vi "DRV_SDSU_reset_ctrler.vi"(0 "fd":i32, 11 "error in (no error)":errorcluster) -> (4 "fd out":i32, 8 "return value":i32, 15 "error out":errorcluster)   [LabVIEW 2016]
doc: "This VI resets the SDSU-II controller."
uses:
  c/lib/libarcDHE.so
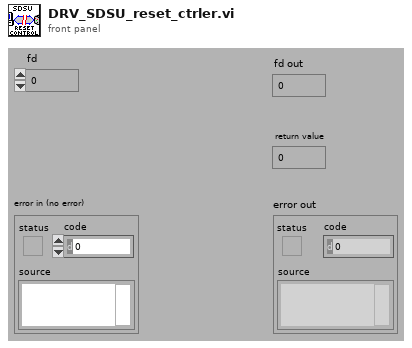
[diagram p1: front panel]
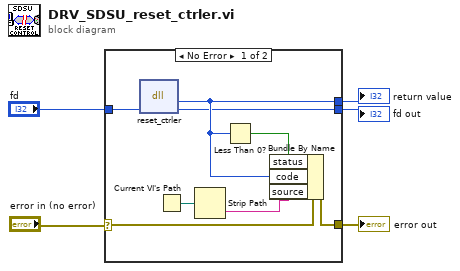
[diagram p0: block diagram]
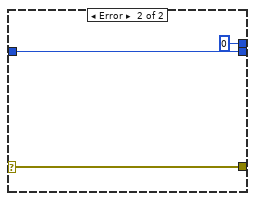
[diagram p2: hidden frame]
diagram:
  n1 = case shown="No Error" "error in (no error)" {
    selector: "error in (no error)" -> [w6 w14]
    tunnel: "fd" -> [w13 w16]
    tunnel: [w11 0] -> w4
    tunnel: [w8 w14] -> w3
    tunnel: [w7 w16] -> w2
    frame No Error {
      n2 = dll-call lib="home/simager/panview/PAN/Modules/SDSU/private/c/lib/libarcDHE.so" fn="reset_ctrler" label="reset_controller"("fd"=w13) -> ("return type"=w11:i32, "fd"=w7:i32)  [unwired: 3 in, 2 out]
      n3 = Current VI's Path() -> (path=w10:path)
      n4 = Strip Path(path=w10) -> (name=w9:string)  [unwired: 1 out]
      n5 = Less Than 0?(x=w11) -> (x < 0?=w12:bool)
      n6 = Bundle By Name(cluster=w6, "status"=w12, "code"=w11, "source"=w9) -> (w8:errorcluster)
    }
    frame Error {
    }
  }
  "error out" <- w3
  "return value" <- w4
  "fd out" <- w2
